vi "update_phase_cal.vi"(11 "Phase errors":sgl[][](array[numeric])) -> ()   [LabVIEW 2011]
uses:
  <vilib>/Analysis/coordinate.llb/Angle Units.ctl
  <vilib>/Analysis/coordinate.llb/Wrap Angle (array).vi
  initialization/globals.vi
  <vilib>/Analysis/NI_AALBase.lvlib
  <vilib>/Analysis/NI_AAL_Angle.lvlib
panel:
  in  "Actually do it":bool=TRUE
  out "New lags":dbl[](array[numeric])
  out "New phase comp":dbl[][](array[numeric])
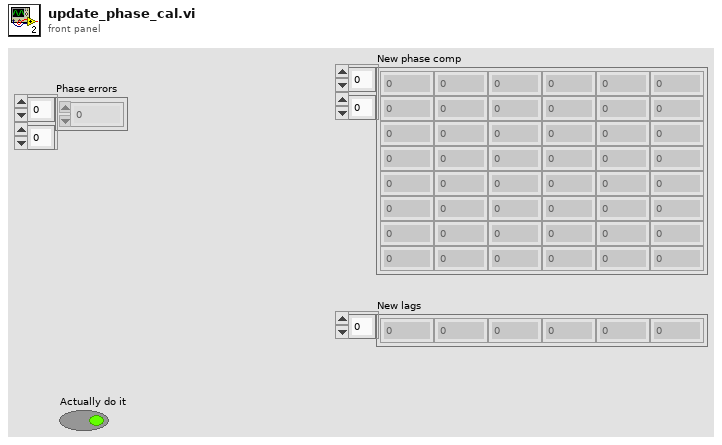
[diagram p1: front panel]
types:
  T1 = typedef "NI_AAL_Angle.lvlib/Angle Units.ctl" = i32
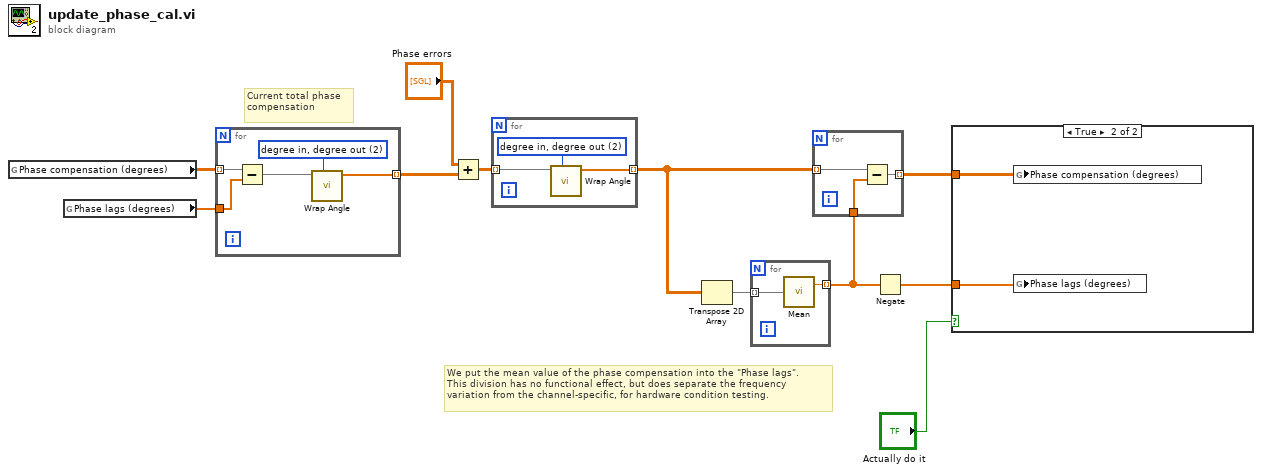
[diagram p0: block diagram]
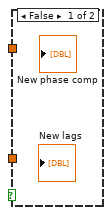
[diagram p2: hidden frame]
diagram:
  # "Current total phase compensation"
  # "We put the mean value of the phase compensation into the \"Phase lags\".\nThis division has no functional effect, but does separate the frequency\nvariation from the channel-specific, for hardware condition testing."
  n1 = global read "globals.vi" "Phase compensation (degrees)"() -> (w10:dbl[][])
  n2 = global read "globals.vi" "Phase lags (degrees)"() -> (w9:dbl[])
  n3 = for {
    tunnel: w10 -> [w16] mode=indexing
    tunnel: w9 -> [w15]
    tunnel: [w12] -> w8 mode=indexing
    w14 = T1 2 items=["radian in, radian out", "radian in, degree out", "degree in, degree out", "degree in, radian out"] ("angle units")
    n4 = Subtract(x=w16, y=w15) -> (x-y=w13:dbl[])
    n5 = call-poly <vilib>:"Wrap Angle.vi"("angle units"=w14, "Angle In"=w13) -> ("Angle Out"=w12:dbl[])  [unwired: 8 in, 1 out]
  }
  n6 = Add(x="Phase errors", y=w8) -> (x+y=w5:dbl[][])
  n7 = for {
    tunnel: w5 -> [w18] mode=indexing
    tunnel: [w17] -> w4 mode=indexing
    w19 = T1 2 items=["radian in, radian out", "radian in, degree out", "degree in, degree out", "degree in, radian out"] ("angle units")
    n8 = call-poly <vilib>:"Wrap Angle.vi"("angle units"=w19, "Angle In"=w18) -> ("Angle Out"=w17:dbl[])  [unwired: 8 in, 1 out]
  }
  n9 = Transpose 2D Array(2D array=w4) -> (transposed array=w11:dbl[][])
  n10 = for {
    tunnel: w11 -> [w21] mode=indexing
    tunnel: [w20] -> w6 mode=indexing
    n11 = call <vilib>:"Mean.vi"("X"=w21) -> ("mean"=w20:dbl)  [unwired: 1 out]
  }
  n12 = for {
    tunnel: [w24] -> w3 mode=indexing
    tunnel: w6 -> [w23]
    tunnel: w4 -> [w22] mode=indexing
    n13 = Subtract(x=w22, y=w23) -> (x-y=w24:dbl[])
  }
  n14 = Negate(x=w6) -> (-x=w2:dbl[])
  n15 = case shown="True" "Actually do it" {
    tunnel: w3 -> [_ w26]
    tunnel: w2 -> [_ w25]
    frame False {
    }
    frame True {
      n16 = global write "globals.vi" "Phase compensation (degrees)"(w26) -> ()
      n17 = global write "globals.vi" "Phase lags (degrees)"(w25) -> ()
    }
  }
